vi "Configure Analog Task Acquisition.vi"(7 "Analog Acquisition Parameters":T1={"sampling frequency Analog"=1000, "number of samples Analog"=1000, "Channels Analog"=[]} {"number of samples Analog" scale=0.0..2000.0; "sampling frequency Analog" scale=0.0..2000.0}, 8 "error in":errorcluster, 9 "Total Acquisition Time":i32, 10 "DAQ Device Name":tag) -> (0 "error out":errorcluster)   [LabVIEW 2020, in "Acquisition.lvlib"]
doc: "Request to configure all the parameters needed for the Analog Acquisition to be realized by its Helper Loop.\n_____\nCreated using Delacor QMH Event Scripter 6.0.0.121."
uses:
  Acquisition.lvlib
  Shared/AnalogAcquisitionParameters__typedef.ctl
  Configure Analog Task Acquisition Argument--cluster.ctl
  Shared/Configuration for Acquisitions.lvlib
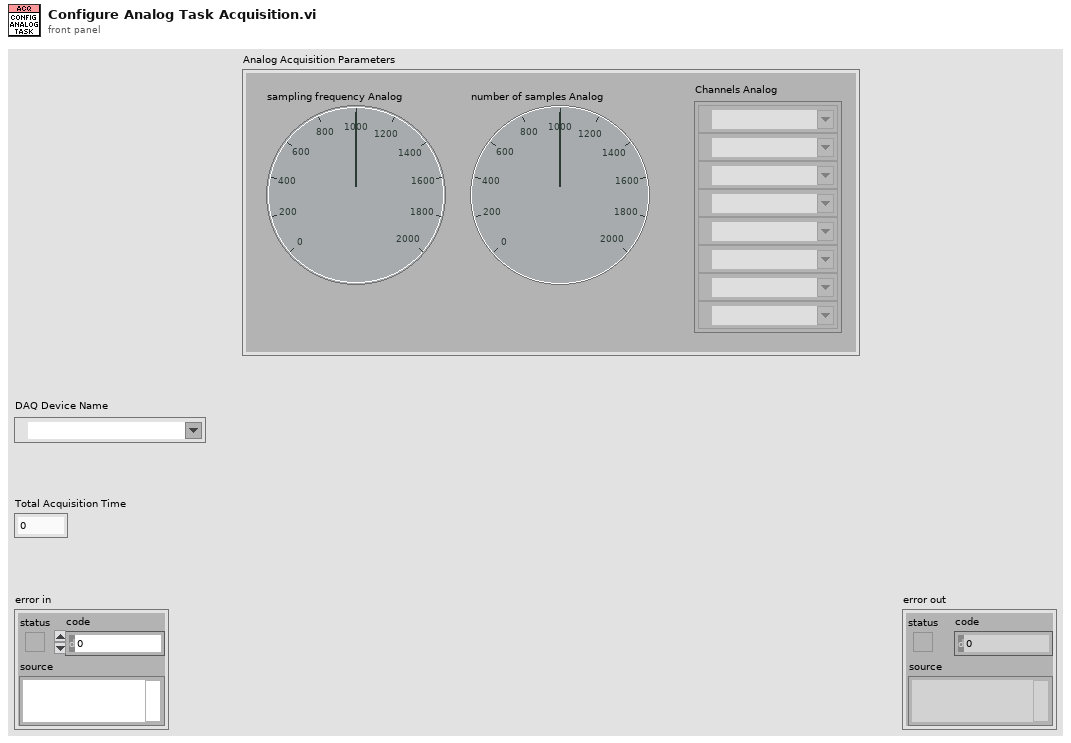
[diagram p1: front panel]
types:
  T1 = typedef "Configuration for Acquisitions.lvlib/AnalogAcquisitionParameters__typedef.ctl" = cluster{"sampling frequency Analog":u32, "number of samples Analog":u32, "Channels Analog":tag[]}
  T2 = typedef "Acquisition.lvlib/Configure Analog Task Acquisition Argument--cluster.ctl" = cluster{"DAQ Device Name":tag, "Total Acquisition Time":i32, "Analog Acquisition Parameters":T1}
  T3 = typedef "Acquisition.lvlib/Request Events--cluster.ctl" = cluster{"Stop Module":refnum<user-event>, "Show Panel":refnum<user-event>, "Hide Panel":refnum<user-event>, "Get Module Execution Status":refnum<user-event>, "Show Diagram":refnum<user-event>, "Start Acquisition":refnum<user-event>, "Configure Analog Task Acquisition":refnum<user-event>, "Configure Digital Taks Acquisition":refnum<user-event>, "Start Analog Acquisition Helper Loop":refnum<user-event>, "Start Digital Acquisition Helper Loop":refnum<user-event>, "Stop Analog Acquisition Helper Loop":refnum<user-event>, "Stop Digital Acquisition Helper Loop":refnum<user-event>}
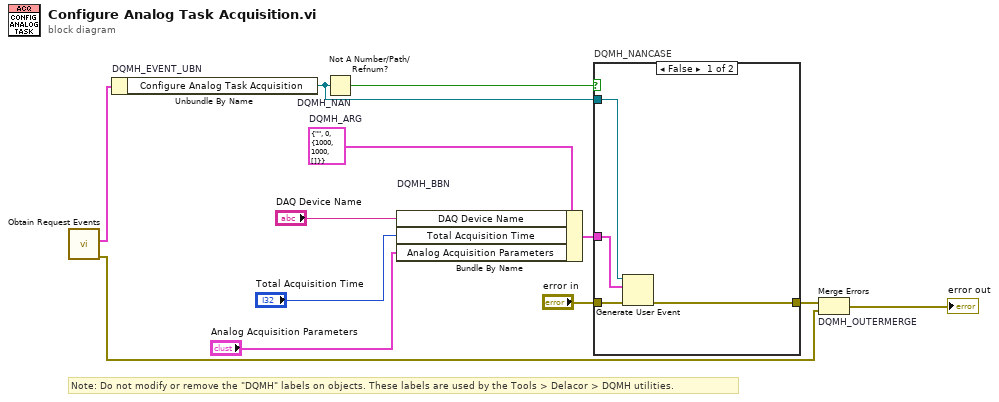
[diagram p0: block diagram]
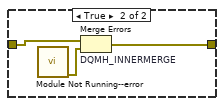
[diagram p2: hidden frame]
diagram:
  w6 = T2 {"DAQ Device Name"="", "Total Acquisition Time"=0, "Analog Acquisition Parameters"={"sampling frequency Analog"=1000, "number of samples Analog"=1000, "Channels Analog"=[]}}  # DQMH_ARG
  # "Note: Do not modify or remove the \"DQMH\" labels on objects. These labels are used by the Tools > Delacor > DQMH utilities."
  n1 = call "Obtain Request Events.vi"() -> ("error out"=w2:errorcluster, "Acquisition Request Events"=w1:T3)  [unwired: 10 in]
  n2 = Unbundle By Name "DQMH_EVENT_UBN"(w1) -> ("Configure Analog Task Acquisition"=w8:refnum<user-event>)
  n3 = Not A Number/Path/Refnum? "DQMH_NAN"(number/path/refnum=w8) -> (NaN/Path/Refnum?=w9:bool)
  n4 = Bundle By Name "DQMH_BBN"(cluster=w6, "DAQ Device Name"="DAQ Device Name", "Total Acquisition Time"="Total Acquisition Time", "Analog Acquisition Parameters"="Analog Acquisition Parameters") -> (w10:T2)
  n5 = case "DQMH_NANCASE" shown="False" w9 {
    tunnel: "error in" -> [w16 w19]
    tunnel: [w15 w18] -> w7
    tunnel: w8 -> [w14 _]
    tunnel: w10 -> [w13 _]
    frame False {
      n6 = Generate User Event(user event=w14, event data cluster=w13, error in=w16) -> (error out=w15:errorcluster)  [unwired: 1 in, 1 out]
    }
    frame True {
      n7 = call "Module Not Running--error.vi"() -> ("error out"=w17:errorcluster)  [unwired: 11 in]
      n8 = Merge Errors "DQMH_INNERMERGE"(w19, w17) -> (w18:errorcluster)
    }
  }
  n9 = Merge Errors "DQMH_OUTERMERGE"(w7, w2) -> (→"error out":errorcluster)
